vi "bigcryo_Harry-IcH - v6.vi"(6 "Mag Field Step":dbl=0.002, 7 "Directory Output":string="C:\\User Data\\gy251\\20210702 AEN017C remeasure in bigcryo\\JJ3\\IcH_pos_to_neg_T=1p6K_set=4p0T", 8 "Stop Field":dbl=-0.1, 9 "Start Field (T)":dbl=0.1 format="%#_7f", 10 "Stop":bool, 11 "Measure":bool) -> ()   [LabVIEW 2019]
uses:
  Components/Global 2.vi
  Components/B_Globals.vi
  <vilib>/Utility/file.llb/Read From Spreadsheet File (DBL).vi
panel:
  out "Sample Temp [K] - Meas":dbl=4.2403
  out "dV/dI-I":cluster{dbl[], dbl[]}(graph) caption="XY Graph"
  out "I-V":cluster{dbl[], dbl[]}(graph) caption="XY Graph"
  out "Status":string="Welcome!"
  in  "Keithley":refnum<visa-resource-name>="GPIB1::20::INSTR"
  in  "Delay [sec]":dbl=0.002 format="%#_6e"
  in  "Compliance [V] 2":dbl=1.0 format="%#_6f"
  in  "Delta [A]":dbl=1e-05 format="%#_6e"
  in  "Abort Conductance":bool
  in  "Step [A]":dbl=1e-05 format="%#_6e"
  in  "I-Max [A]":dbl=0.002 format="%#_6e"
  in  "Arm Conductance":bool
  out "B Now":string="-0.101"
  out "error out 6":errorcluster
  in  "Minicryo":bool=TRUE
  in  "Field and rate":dbl[][](array[numeric])
  in  "step":bool=TRUE
  in  "Set Rate (T/min)":dbl=0.05
  out "?":refnum<visa-resource-name>="GPIB1::20::INSTR"
  out "Iteration?":i32=1001
  out "Path Out":path=path "C:/User Data/hlb54/gigi.dat"
  out "B Aim":dbl=-0.101
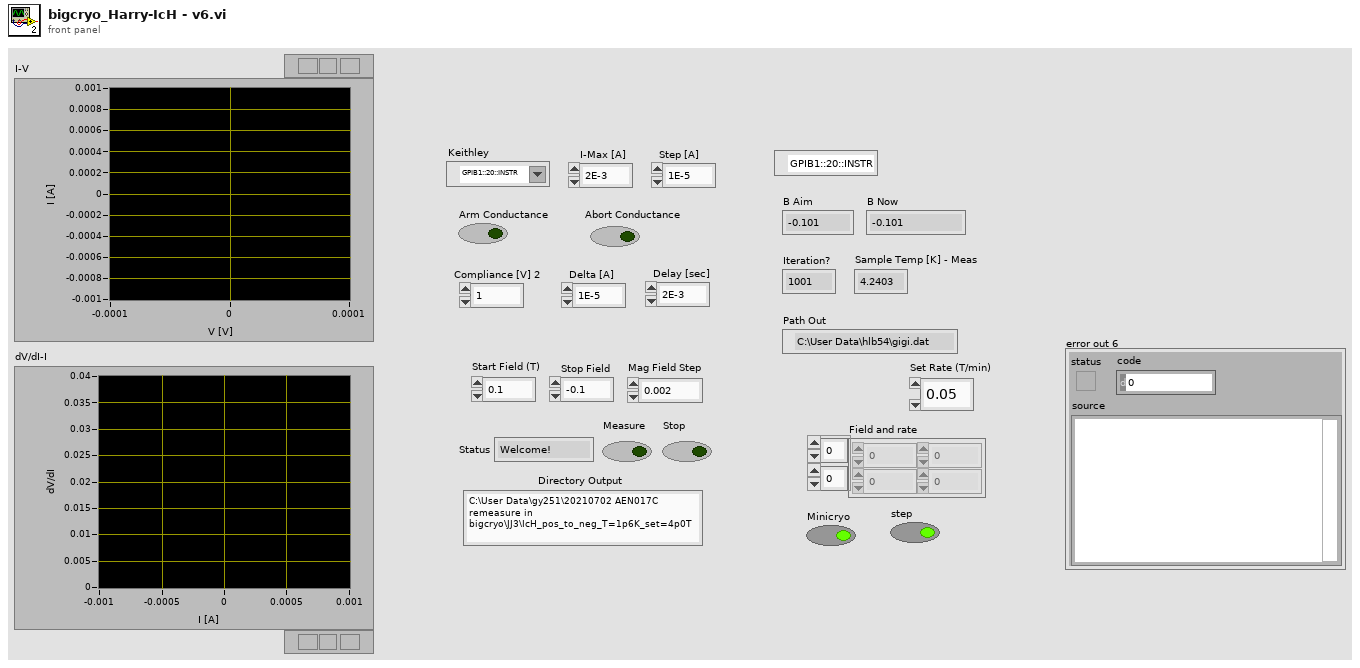
[diagram p1: front panel]
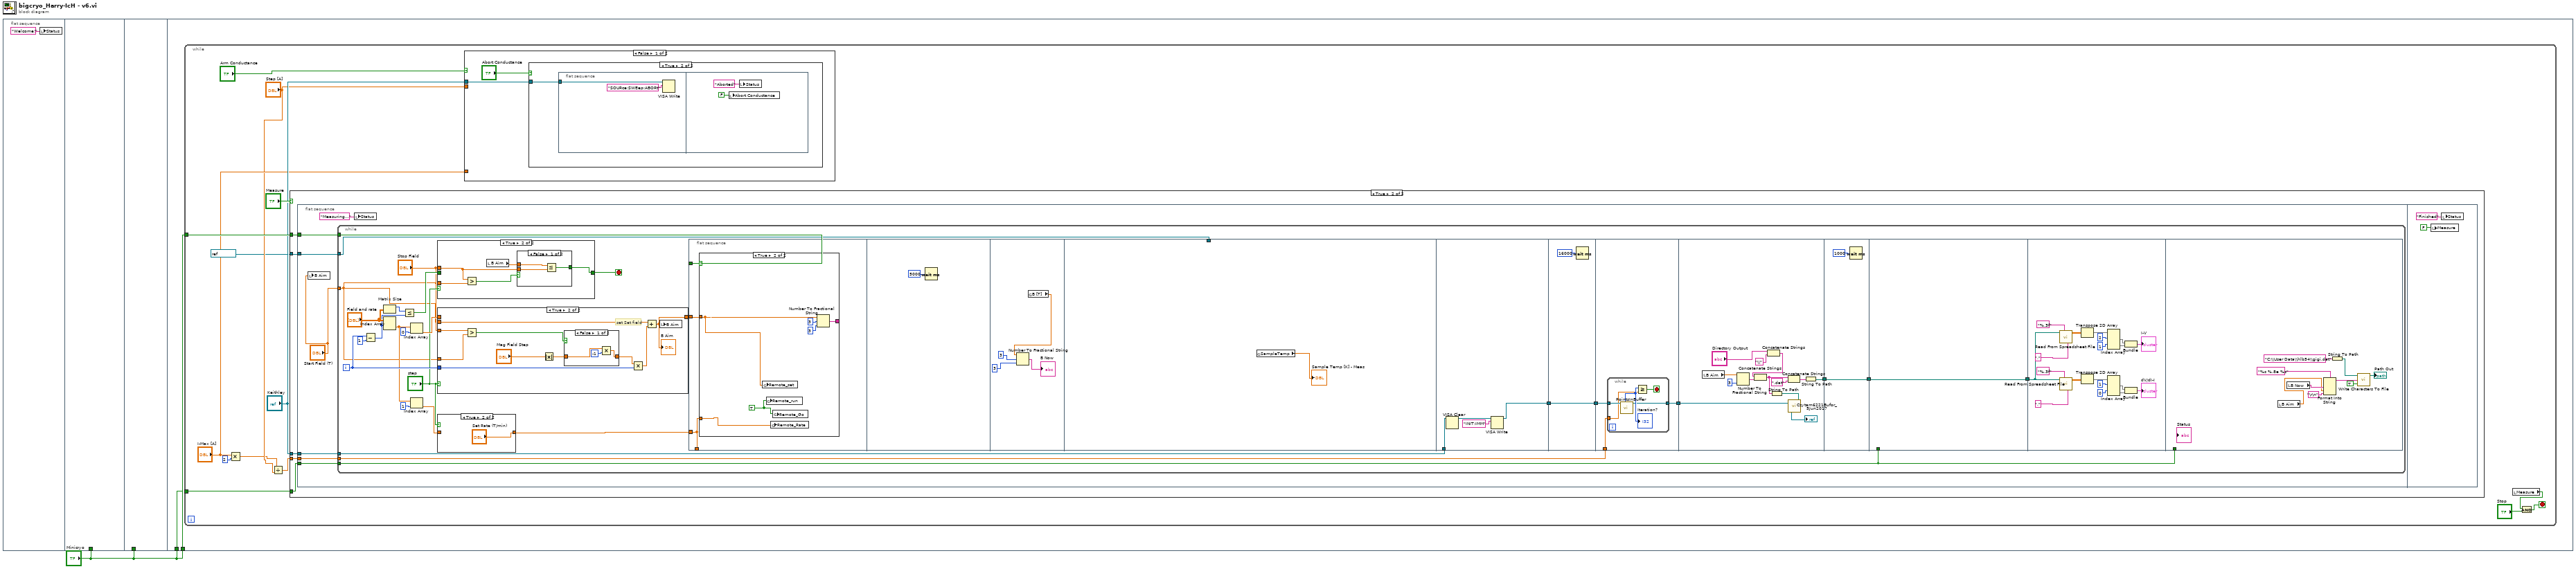
[diagram p0: block diagram]
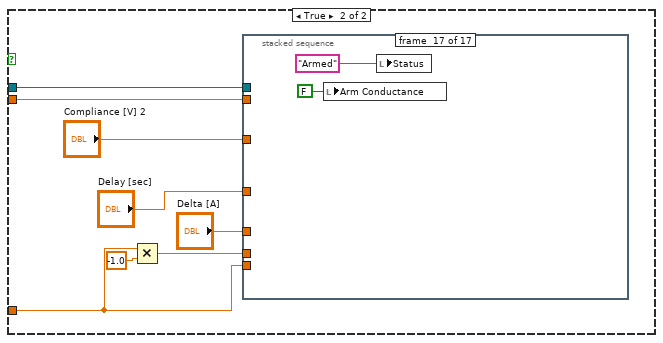
[diagram p3: hidden frame]
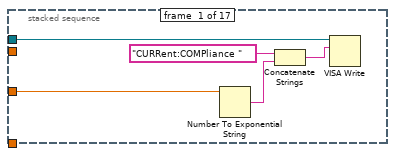
[diagram p4: hidden frame]
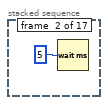
[diagram p5: hidden frame]
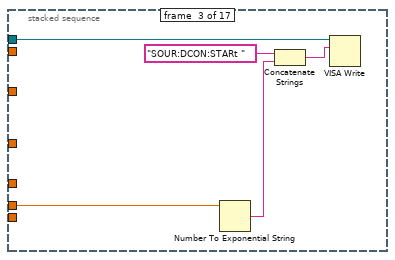
[diagram p6: hidden frame]
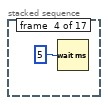
[diagram p7: hidden frame]
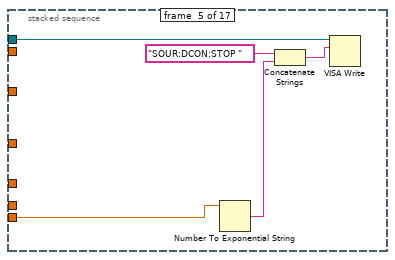
[diagram p8: hidden frame]
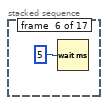
[diagram p9: hidden frame]
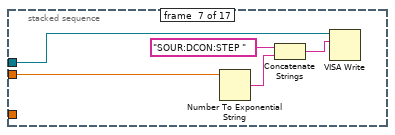
[diagram p10: hidden frame]
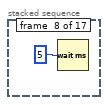
[diagram p11: hidden frame]
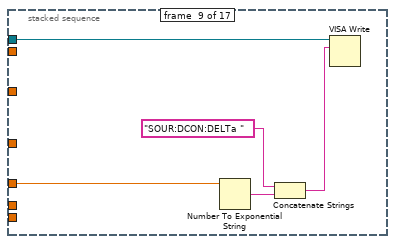
[diagram p12: hidden frame]
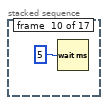
[diagram p13: hidden frame]
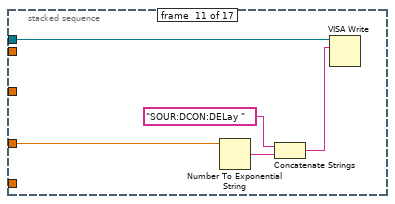
[diagram p14: hidden frame]
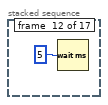
[diagram p15: hidden frame]
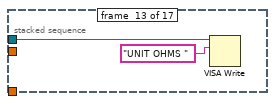
[diagram p16: hidden frame]
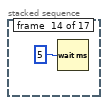
[diagram p17: hidden frame]
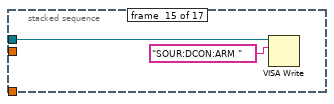
[diagram p18: hidden frame]
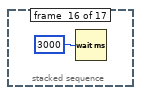
[diagram p19: hidden frame]
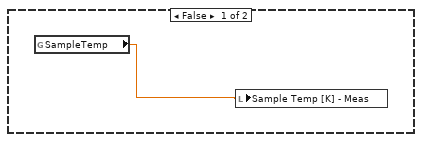
[diagram p20: hidden frame]
diagram:
  n1 = flat-sequence {
    tunnel: "Minicryo" -> [_]
    tunnel: "Minicryo" -> [_]
    tunnel: "Minicryo" -> [w4]
    tunnel: "Minicryo" -> [w3]
    frame #0 {
      n2 = local write "Status"("Welcome!") -> ()
    }
    frame #1 {
    }
    frame #2 {
    }
    frame #3 {
      n3 = while {
        tunnel: w4 -> [w18]
        tunnel: w3 -> [w17]
        stop <- w6 stop-if-true
        n4 = Multiply(x="I-Max [A]", y=2) -> (x*y=w9:dbl)
        n5 = Divide(x=w9, y="Step [A]") -> (x/y=w10:dbl)
        n6 = case shown="True" "Measure" {
          tunnel: w18 -> [_ w83]
          tunnel: w17 -> [_ w82]
          tunnel: "Keithley" -> [_ w81]
          tunnel: w10 -> [_ w80]
          tunnel: refnum<visa-resource-name> "COM7" ("LakeShore340") -> [_ w79]
          frame False {
            n7 = global read "Global 2.vi" "SampleTemp"() -> (w78:dbl)
            n8 = local write "Sample Temp [K] - Meas"(w78) -> ()
          }
          frame True {
            n9 = flat-sequence {
              tunnel: w83 -> [w90]
              tunnel: w82 -> [w89]
              tunnel: w81 -> [w88]
              tunnel: w80 -> [w87]
              tunnel: w79 -> [w85]
              frame #0 {
                n10 = local write "B Aim"("Start Field (T)") -> ()
                n11 = while {
                  tunnel: w90 -> [w106]
                  tunnel: w89 -> [w101]
                  tunnel: w88 -> [w99]
                  tunnel: w87 -> [w98]
                  tunnel: w85 -> [w92]
                  tunnel: "Start Field (T)" -> [w91]
                  i -> [w112]
                  stop <- w97 stop-if-true
                  n12 = Subtract(x=w112, y=1) -> (x-y=w103:i32)
                  n13 = Matrix Size(0:"Field and rate") -> (1:w104:i32)  [unwired: 1 out]
                  n14 = Index Array(array="Field and rate", index (row)=w103) -> (element=w109:dbl[])  [unwired: 1 in]
                  n15 = Less Or Equal?(x=w104, y=w103) -> (x <= y?=w102:bool)
                  n16 = Index Array(array=w109, index=0) -> (element=w108:dbl)
                  n17 = Index Array(array=w109, index=1) -> (element=w107:dbl)
                  n18 = case shown="True" "step" {
                    tunnel: [w119 w124] -> w97
                    tunnel: w102 -> [w119 _]
                    tunnel: "Stop Field" -> [_ w122]
                    tunnel: w91 -> [_ w121]
                    frame False {
                    }
                    frame True {
                      n19 = Greater?(x=w122, y=w121) -> (0:w120:bool)
                      n20 = local read "B Aim"() -> (w123:dbl)
                      n21 = case shown="False" w120 {
                        tunnel: [w127 w130] -> w124
                        tunnel: w123 -> [w125 w129]
                        tunnel: w122 -> [w126 w128]
                        frame False {
                          n22 = Less Or Equal?(x=w125, y=w126) -> (x <= y?=w127:bool)
                        }
                        frame True {
                          n23 = Greater Or Equal?(x=w129, y=w128) -> (x >= y?=w130:bool)
                        }
                      }
                    }
                  }
                  n24 = case shown="True" "step" {
                    tunnel: [w133 w142] -> w118
                    tunnel: w112 -> [_ w141]
                    tunnel: w108 -> [w133 _]
                    tunnel: w91 -> [_ w140]
                    tunnel: w91 -> [_ w139]
                    tunnel: "Stop Field" -> [_ w138]
                    frame False {
                    }
                    frame True {
                      # "set Set field"
                      n25 = Greater?(x=w138, y=w139) -> (0:w134:bool)
                      n26 = Absolute Value(x="Mag Field Step") -> (abs(x)=w136:dbl)
                      n27 = case shown="False" w134 {
                        tunnel: [w146 w147] -> w135
                        tunnel: w136 -> [w144 w147]
                        frame False {
                          n28 = Multiply(x=w144, y=-1) -> (x*y=w146:dbl)
                        }
                        frame True {
                        }
                      }
                      n29 = Multiply(x=w135, y=w141) -> (x*y=w143:dbl)
                      n30 = Add(x=w140, y=w143) -> (x+y=w142:dbl)
                      "B Aim" <- w142
                      n31 = local write "B Aim"(w142) -> ()
                    }
                  }
                  n32 = case shown="True" "step" {
                    tunnel: [w131 "Set Rate (T/min)"] -> w114
                    tunnel: w107 -> [w131 _]
                    frame False {
                    }
                    frame True {
                    }
                  }
                  n33 = flat-sequence {
                    tunnel: w118 -> [w150]
                    tunnel: [w149] -> _
                    tunnel: w114 -> [w149]
                    tunnel: w106 -> [w148]
                    tunnel: w92 -> [_]
                    tunnel: [w173] -> w116
                    tunnel: w99 -> [w172]
                    tunnel: [w177] -> w117
                    tunnel: w116 -> [w177]
                    tunnel: w117 -> [w180]
                    tunnel: [w179] -> w115
                    tunnel: w98 -> [w178]
                    tunnel: w115 -> [w193]
                    tunnel: [w189] -> w93
                    tunnel: [w199] -> w94
                    tunnel: w93 -> [w199]
                    tunnel: w101 -> [_]
                    tunnel: [w201] -> w95
                    tunnel: w94 -> [w201]
                    tunnel: w95 -> [w202]
                    tunnel: w101 -> [_]
                    frame #0 {
                      n34 = case shown="True" w148 {
                        tunnel: w150 -> [w153 w160]
                        tunnel: w149 -> [_ w162]
                        tunnel: [w151 w163] -> _
                        frame False {
                          n35 = Number To Fractional String(number=w153, width (-)=i16 3, precision (6)=i16 3) -> (F-format string=w151:string)  [unwired: 1 in]
                          n36 = Concatenate Strings("J" ("string"), w151) -> (w152:string)
                          n37 = GPIB Write(0:"25" ("address string"), 1:w152, 2:6) -> (6:→"error out 6":errorcluster)  [unwired: 2 in, 1 out]
                        }
                        frame True {
                          w161 = TRUE
                          n38 = global write "B_Globals.vi" "Remote_set"(w160) -> ()
                          n39 = global write "B_Globals.vi" "Remote_run"(w161) -> ()
                          n40 = global write "B_Globals.vi" "Remote_Rate"(w162) -> ()
                          n41 = global write "B_Globals.vi" "Remote_Go"(w161) -> ()
                          n42 = Number To Fractional String(number=w160, width (-)=i16 3, precision (6)=i16 3) -> (F-format string=w163:string)  [unwired: 1 in]
                        }
                      }
                    }
                    frame #1 {
                      n43 = Wait (ms)(milliseconds to wait=u32 5000) -> ()  [unwired: 1 out]
                    }
                    frame #2 {
                      n44 = global read "B_Globals.vi" "B [T]"() -> (w167:dbl)
                      n45 = Number To Fractional String(number=w167, width (-)=i16 3, precision (6)=i16 3) -> (F-format string=→"B Now":string)  [unwired: 1 in]
                    }
                    frame #3 {
                      n46 = global read "Global 2.vi" "SampleTemp"() -> (→"Sample Temp [K] - Meas":dbl)
                    }
                    frame #4 {
                      n47 = VISA Clear(VISA resource name=w172) -> (VISA resource name out=w175:refnum<visa-resource-name>)  [unwired: 1 in, 1 out]
                      n48 = VISA Write(VISA resource name=w175, write buffer="INIT:IMM") -> (VISA resource name out=w173:refnum<visa-resource-name>)  [unwired: 1 in, 2 out]
                    }
                    frame #5 {
                      n49 = Wait (ms)(milliseconds to wait=16000) -> ()  [unwired: 1 out]
                    }
                    frame #6 {
                      n50 = while {
                        tunnel: w180 -> [w183]
                        tunnel: [w182] -> w179
                        tunnel: w178 -> [w181]
                        stop <- w184 stop-if-true
                        n51 = call "PointsInBuffer.vi"("VISA resource name"=w183) -> (3:w182:refnum<visa-resource-name>, "number"=w185:i32)  [unwired: 9 in]
                        "Iteration?" <- w185
                        n52 = Greater Or Equal?(x=w185, y=w181) -> (x >= y?=w184:bool)
                      }
                    }
                    frame #7 {
                      n53 = local read "B Aim"() -> (w194:dbl)
                      n54 = Number To Fractional String(number=w194, precision (6)=i16 3) -> (F-format string=w198:string)  [unwired: 2 in]
                      n55 = Concatenate Strings("Directory Output", "\\") -> (w186:string)
                      n56 = Concatenate Strings(w186, w198) -> (w191:string)
                      n57 = String To Path(string=w191) -> (path=w197:path)
                      n58 = Concatenate Strings(w191, ".dat") -> (w190:string)
                      n59 = call "Czytam6221Bufor_5Jun2017.vi"("file path (dialog if empty)"=w197, 3:w193) -> (2:→"?":refnum<visa-resource-name>)  [unwired: 1 in]
                      n60 = String To Path(string=w190) -> (path=w189:path)
                    }
                    frame #8 {
                      n61 = Wait (ms)(milliseconds to wait=u32 1000) -> ()  [unwired: 1 out]
                    }
                    frame #9 {
                    }
                    frame #10 {
                      n62 = call-poly <vilib>:"Read From Spreadsheet File.vi"("delimiter (\\t)"="," ("delimiter (\\t)"), "format (%.3f)"="%.3f", "file path (dialog if empty)"=w202) -> ("all rows"=w215:dbl[][])  [unwired: 4 in, 4 out]
                      n63 = call-poly <vilib>:"Read From Spreadsheet File.vi"("delimiter (\\t)"="," ("delimiter (\\t)"), "format (%.3f)"="%.3f", "file path (dialog if empty)"=w202) -> ("all rows"=w206:dbl[][])  [unwired: 4 in, 4 out]
                      n64 = Transpose 2D Array(2D array=w215) -> (transposed array=w214:dbl[][])
                      n65 = Transpose 2D Array(2D array=w206) -> (transposed array=w205:dbl[][])
                      n66 = Index Array(array=w214, index (row) #1=2 ("index (row)"), index (row) #2=1 ("index (row)")) -> (element #1=w217:dbl[], element #2=w216:dbl[])  [unwired: 2 in]
                      n67 = Index Array(array=w205, index (row) #1=1 ("index (row)"), index (row) #2=0 ("index (row)")) -> (element #1=w208:dbl[], element #2=w207:dbl[])  [unwired: 2 in]
                      n68 = Bundle(w217, w216) -> (→"I-V":cluster{dbl[], dbl[]})  [unwired: 1 in]
                      n69 = Bundle(w208, w207) -> (→"dV/dI-I":cluster{dbl[], dbl[]})  [unwired: 1 in]
                    }
                    frame #11 {
                      n70 = local read "B Aim"() -> (w221:dbl)
                      n71 = local read "B Now"() -> (w224:string)
                      n72 = Format Into String(format string="%s %.8e %s", w224, w221, "\r\n") -> (resulting string=w227:string)  [unwired: 2 in, 1 out]
                      n73 = String To Path(string="C:\\User Data\\hlb54\\gigi.dat") -> (path=w222:path)
                      n74 = call <vilib>:"Write Characters To File.vi"("append to file? (new file:F)"=TRUE, "character string"=w227, "file path (dialog if empty)"=w222) -> ("new file path (Not A Path if cancelled)"=→"Path Out":path)  [unwired: 2 out]
                    }
                  }
                }
                n75 = local write "Status"("Measuring...") -> ()
              }
              frame #1 {
                n76 = local write "Measure"(FALSE) -> ()
                n77 = local write "Status"("Finished") -> ()
              }
            }
          }
        }
        n78 = case shown="False" "Arm Conductance" {
          tunnel: "Keithley" -> [w19 w29]
          tunnel: "Step [A]" -> [_ w28]
          tunnel: "I-Max [A]" -> [_ w26]
          frame False {
            n79 = case shown="True" "Abort Conductance" {
              tunnel: w19 -> [_ w21]
              frame False {
              }
              frame True {
                n80 = flat-sequence {
                  tunnel: w21 -> [w22]
                  frame #0 {
                    n81 = VISA Write(VISA resource name=w22, write buffer="SOURce:SWEep:ABORt") -> ()  [unwired: 1 in, 3 out]
                  }
                  frame #1 {
                    n82 = local write "Abort Conductance"(FALSE) -> ()
                    n83 = local write "Status"("Aborted") -> ()
                  }
                }
              }
            }
          }
          frame True {
            n84 = Multiply(x=w26, y=-1.0) -> (x*y=w27:dbl)
            n85 = stacked-sequence {
              tunnel: w27 -> [_ _ w42 _ _ _ _ _ _ _ _ _ _ _ _ _ _]
              tunnel: "Delay [sec]" -> [_ _ _ _ _ _ _ _ _ _ w65 _ _ _ _ _ _]
              tunnel: "Compliance [V] 2" -> [w35 _ _ _ _ _ _ _ _ _ _ _ _ _ _ _ _]
              tunnel: "Delta [A]" -> [_ _ _ _ _ _ _ _ w59 _ _ _ _ _ _ _ _]
              tunnel: w29 -> [w34 _ w40 _ w47 _ w53 _ w58 _ w64 _ w70 _ w73 _ _]
              tunnel: w28 -> [_ _ _ _ _ _ w52 _ _ _ _ _ _ _ _ _ _]
              tunnel: w26 -> [_ _ _ _ w46 _ _ _ _ _ _ _ _ _ _ _ _]
              frame #0 {
                n86 = Number To Exponential String(number=w35) -> (E-format string=w37:string)  [unwired: 3 in]
                n87 = Concatenate Strings("CURRent:COMPliance ", w37) -> (w36:string)
                n88 = VISA Write(VISA resource name=w34, write buffer=w36) -> ()  [unwired: 1 in, 3 out]
              }
              frame #1 {
                n89 = Wait (ms)(milliseconds to wait=5) -> ()  [unwired: 1 out]
              }
              frame #2 {
                n90 = Number To Exponential String(number=w42) -> (E-format string=w43:string)  [unwired: 3 in]
                n91 = Concatenate Strings("SOUR:DCON:STARt ", w43) -> (w41:string)
                n92 = VISA Write(VISA resource name=w40, write buffer=w41) -> ()  [unwired: 1 in, 3 out]
              }
              frame #3 {
                n93 = Wait (ms)(milliseconds to wait=5) -> ()  [unwired: 1 out]
              }
              frame #4 {
                n94 = Number To Exponential String(number=w46) -> (E-format string=w49:string)  [unwired: 3 in]
                n95 = Concatenate Strings("SOUR:DCON:STOP ", w49) -> (w48:string)
                n96 = VISA Write(VISA resource name=w47, write buffer=w48) -> ()  [unwired: 1 in, 3 out]
              }
              frame #5 {
                n97 = Wait (ms)(milliseconds to wait=5) -> ()  [unwired: 1 out]
              }
              frame #6 {
                n98 = Number To Exponential String(number=w52) -> (E-format string=w55:string)  [unwired: 3 in]
                n99 = Concatenate Strings("SOUR:DCON:STEP ", w55) -> (w54:string)
                n100 = VISA Write(VISA resource name=w53, write buffer=w54) -> ()  [unwired: 1 in, 3 out]
              }
              frame #7 {
                n101 = Wait (ms)(milliseconds to wait=5) -> ()  [unwired: 1 out]
              }
              frame #8 {
                n102 = Number To Exponential String(number=w59) -> (E-format string=w61:string)  [unwired: 3 in]
                n103 = Concatenate Strings("SOUR:DCON:DELTa ", w61) -> (w60:string)
                n104 = VISA Write(VISA resource name=w58, write buffer=w60) -> ()  [unwired: 1 in, 3 out]
              }
              frame #9 {
                n105 = Wait (ms)(milliseconds to wait=5) -> ()  [unwired: 1 out]
              }
              frame #10 {
                n106 = Number To Exponential String(number=w65) -> (E-format string=w67:string)  [unwired: 3 in]
                n107 = Concatenate Strings("SOUR:DCON:DELay ", w67) -> (w66:string)
                n108 = VISA Write(VISA resource name=w64, write buffer=w66) -> ()  [unwired: 1 in, 3 out]
              }
              frame #11 {
                n109 = Wait (ms)(milliseconds to wait=5) -> ()  [unwired: 1 out]
              }
              frame #12 {
                n110 = VISA Write(VISA resource name=w70, write buffer="UNIT OHMS ") -> ()  [unwired: 1 in, 3 out]
              }
              frame #13 {
                n111 = Wait (ms)(milliseconds to wait=5) -> ()  [unwired: 1 out]
              }
              frame #14 {
                n112 = VISA Write(VISA resource name=w73, write buffer="SOUR:DCON:ARM ") -> ()  [unwired: 1 in, 3 out]
              }
              frame #15 {
                n113 = Wait (ms)(milliseconds to wait=3000) -> ()  [unwired: 1 out]
              }
              frame #16 {
                n114 = local write "Arm Conductance"(FALSE) -> ()
                n115 = local write "Status"("Armed") -> ()
              }
            }
          }
        }
        n116 = local read "Measure"() -> (w7:bool)
        n117 = And(x=w7, y="Stop") -> (x .and. y?=w6:bool)
      }
    }
  }
